vi "FGVtime.vi"(8 "error in (no error)":errorcluster, 11 "Enum":enum16{"get", "start"}(ring)) -> (0 "error out":errorcluster, 3 "Numeric":dbl)   [LabVIEW 2021]
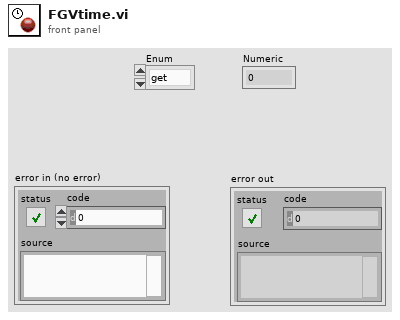
[diagram p1: front panel]
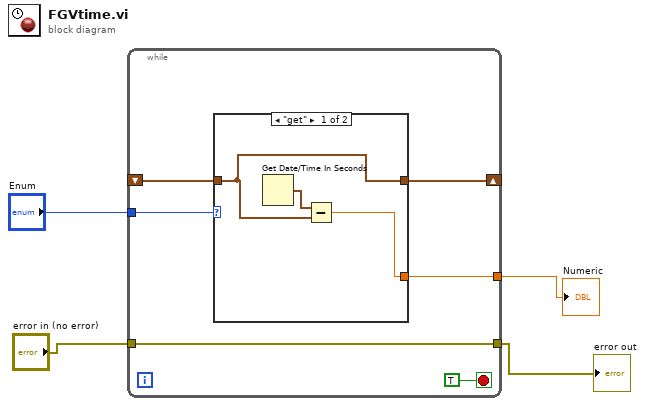
[diagram p0: block diagram]
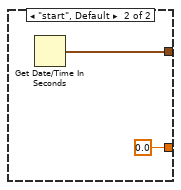
[diagram p2: hidden frame]
diagram:
  n1 = while {
    tunnel: "Enum" -> [w10]
    shift-right: [w9] -> _
    shift-left: _ -> [w7]
    tunnel: [w8] -> w3
    tunnel: [w5] -> w1
    tunnel: "error in (no error)" -> [w5]
    stop <- TRUE stop-if-true
    n2 = case shown="\"get\"" w10 {
      tunnel: [w11 w15] -> w9
      tunnel: [w12 0.0 ("Numeric")] -> w8
      tunnel: w7 -> [w11 _]
      frame "get" {
        n3 = Get Date/Time In Seconds() -> (seconds since 1Jan1904=w13:timestamp)
        n4 = Subtract(x=w13, y=w11) -> (x-y=w12:dbl)
      }
      frame "start", Default {
        n5 = Get Date/Time In Seconds() -> (seconds since 1Jan1904=w15:timestamp)
      }
    }
  }
  "Numeric" <- w3
  "error out" <- w1
